vi "issueCommandExit.vi"(8 "error in (no error)":errorcluster, 11 "SALCommunicatorTC in":refnum<class "SALCommunicatorTC.lvclass">) -> (0 "error out":errorcluster, 3 "SALCommunicatorTC out":refnum<class "SALCommunicatorTC.lvclass">)   [LabVIEW 2016, in "SALCommunicatorTC.lvclass"]
uses:
  SALCommunicatorTC.lvclass
  ts_sallv_exa/DataTypes/command_exitControl.ctl
  ts_sallv_exa/SALLV_EXA.lvlib
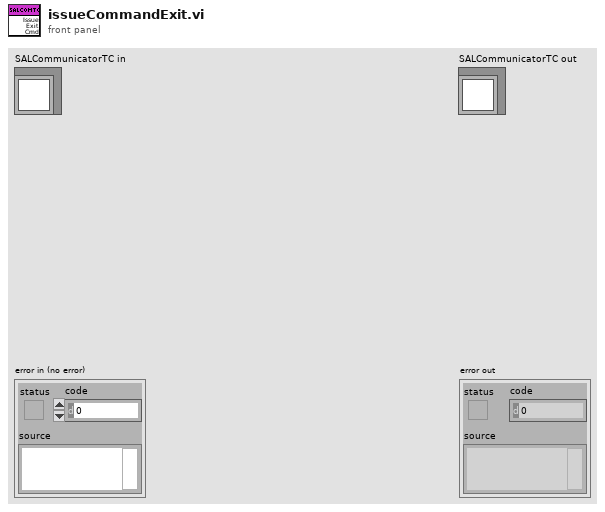
[diagram p1: front panel]
types:
  T1 = typedef "SALLV_EXA.lvlib/command_exitControl.ctl" = cluster{"state":bool}
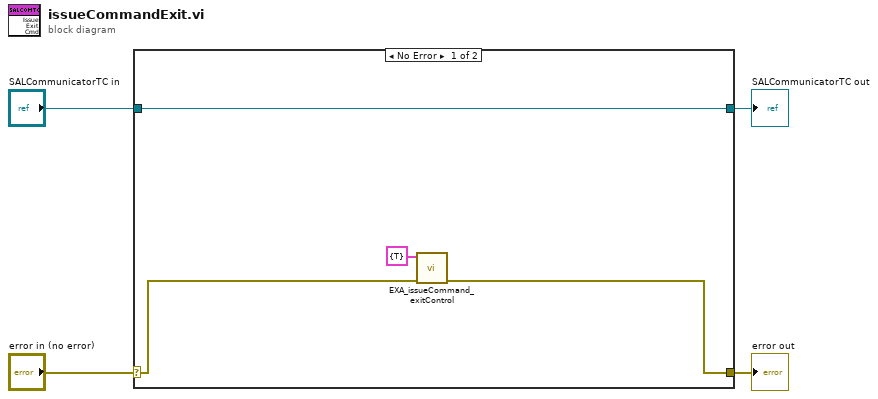
[diagram p0: block diagram]
diagram:
  n1 = case shown="No Error" "error in (no error)" {
    selector: "error in (no error)" -> [w7 w10]
    tunnel: [w6 w10] -> w3
    tunnel: [w8 w9] -> w1
    tunnel: "SALCommunicatorTC in" -> [w8 w9]
    frame No Error {
      n2 = call "EXA_issueCommand_exitControl.vi"("error in (no error)"=w7, "command_exitControl_Ctl"=T1 {"state"=TRUE}) -> ("error out"=w6:errorcluster)  [unwired: 7 in, 2 out]
    }
    frame Error {
    }
  }
  "error out" <- w3
  "SALCommunicatorTC out" <- w1
